vi "Function_generator.vi"() -> ()   [LabVIEW 2020]
uses:
  <vilib>/Instr/_visa.llb/VISA Configure Serial Port (Instr).vi
  <vilib>/measure/NI_MABase.lvlib
panel:
  in  "Sampling Period ( ms )":u32=1000
  in  "Enum":enum16{"Sine", "Square", "Triangle"}(ring)
  out "decimal integer string":string
  out "element":dbl
  in  "VISA resource name":refnum<visa-resource-name>
  out "Waveform Graph":waveform(dbl)(graph)
  in  "frequency":dbl(slide)=10.0 scale=0.0..50.0
  out "Analog":dbl
  in  "stop":bool
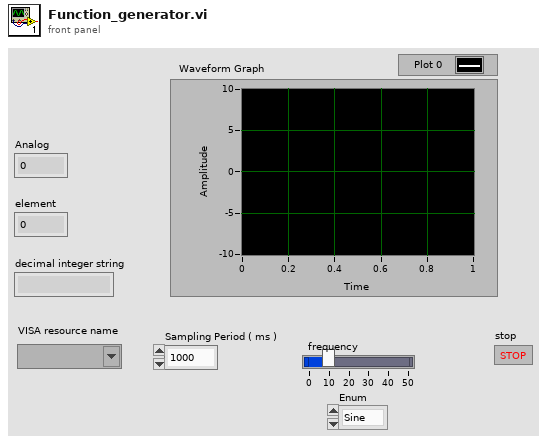
[diagram p1: front panel]
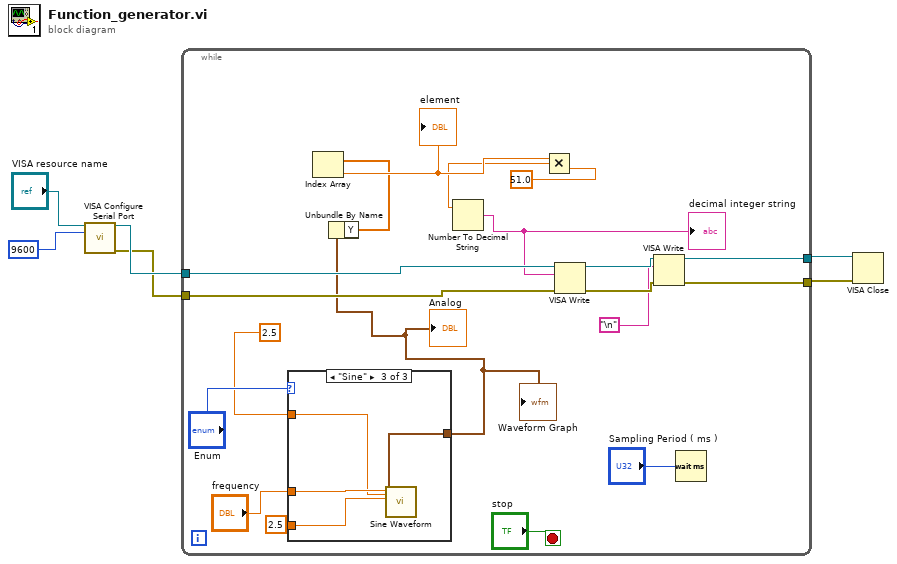
[diagram p0: block diagram]
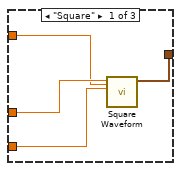
[diagram p2: hidden frame]
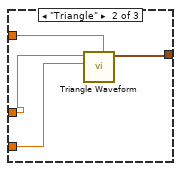
[diagram p3: hidden frame]
diagram:
  n1 = call-poly "VISA Configure Serial Port"("VISA resource name"="VISA resource name", "baud rate (9600)"=u32 9600) -> ("VISA resource name out"=w4:refnum<visa-resource-name>, "error out"=w3:errorcluster)  [unwired: 12 in]
  n2 = while {
    tunnel: w4 -> [w24]
    tunnel: w3 -> [w23]
    tunnel: [w17] -> w2
    tunnel: [w15] -> w1
    stop <- "stop" stop-if-true
    n3 = case shown="\"Sine\"" "Enum" {
      tunnel: "frequency" -> [w29 w33 w37]
      tunnel: [w28 w32 w36] -> w9
      tunnel: 2.5 -> [w27 w31 w35]
      tunnel: 2.5 -> [w26 w30 w34]
      frame "Square" {
        n4 = call <vilib>:"Square Waveform.vi"("offset"=w27, "amplitude"=w26, "frequency"=w29) -> ("signal out"=w28:waveform(dbl))  [unwired: 7 in, 1 out]
      }
      frame "Triangle" {
        n5 = call <vilib>:"Triangle Waveform.vi"("offset"=w31, "amplitude"=w30, "frequency"=w33) -> ("signal out"=w32:waveform(dbl))  [unwired: 7 in, 1 out]
      }
      frame "Sine" {
        n6 = call <vilib>:"Sine Waveform.vi"("offset"=w35, "amplitude"=w34, "frequency"=w37) -> ("signal out"=w36:waveform(dbl))  [unwired: 7 in, 1 out]
      }
    }
    "Analog" <- w9
    "Waveform Graph" <- w9
    n7 = Unbundle By Name(w9) -> ("Y"=w10:dbl[])
    n8 = Index Array(array=w10) -> (element=w22:dbl)  [unwired: 1 in]
    "element" <- w22
    n9 = Multiply(x=w22, y=51.0) -> (x*y=w20:dbl)
    n10 = Number To Decimal String(number=w20) -> (decimal integer string=w19:string)  [unwired: 1 in]
    "decimal integer string" <- w19
    n11 = VISA Write(VISA resource name=w24, write buffer=w19, error in (no error)=w23) -> (VISA resource name out=w18:refnum<visa-resource-name>, error out=w16:errorcluster)  [unwired: 1 out]
    n12 = VISA Write(VISA resource name=w18, write buffer="\n", error in (no error)=w16) -> (VISA resource name out=w17:refnum<visa-resource-name>, error out=w15:errorcluster)  [unwired: 1 out]
    n13 = Wait (ms)(milliseconds to wait="Sampling Period ( ms )") -> ()  [unwired: 1 out]
  }
  n14 = VISA Close(VISA resource name=w2, error in (no error)=w1) -> ()  [unwired: 1 out]
